vi "HHMI - Count U16 old.vi"(7 "Reset?":bool, 10 "Increment?":bool) -> (2 "total # counted\n(Reset occurs \nprior to Increment)":u16)   [LabVIEW 2013]
doc: "Counts up. Reset returns count to zero. Increment occurs after Reset."
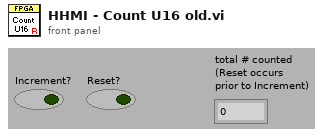
[diagram p1: front panel]
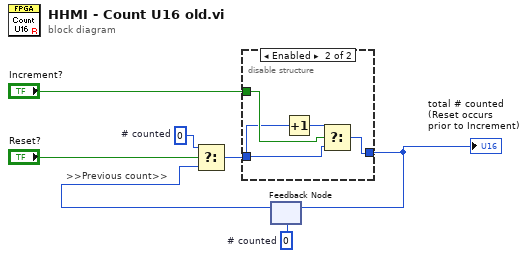
[diagram p0: block diagram]
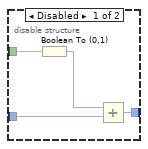
[diagram p2: hidden frame]
diagram:
  w4 = u16 0  # # counted
  w7 = u16 0  # # counted
  # ">>Previous count>>"
  n1 = feedback #1(w7) -> (w5:u16)
  n2 = Select(t=w4, s="Reset?", f=w5) -> (s? t:f=w2:u16)
  n3 = disable-structure shown="Enabled" {
    disable-tunnel: "Increment?" -> [w11 w14]
    disable-tunnel: w2 -> [w10 w13]
    disable-tunnel: [w8 w12] -> w1
    frame Disabled {
      n4 = Boolean To (0,1)(Boolean=w11) -> (0, 1=w9:i16)
      n5 = Add(x=w9, y=w10) -> (x+y=w8:u16)
    }
    frame Enabled {
      n6 = Increment(x=w13) -> (x+1=w15:u16)
      n7 = Select(t=w15, s=w14, f=w13) -> (s? t:f=w12:u16)
    }
  }
  "total # counted\n(Reset occurs \nprior to Increment)" <- w1
  n8 = feedback-in #1(w1) -> ()
